vi "Straight line spline generator.vi"(10 "Y":dbl format="%#_13g", 11 "X":dbl format="%#_13g") -> (2 "bx^3":dbl, 3 "ax^3":dbl)   [LabVIEW 2015]
uses:
  <vilib>/Analysis/7linalg.llb/Solve Linear Equations (single right hand).vi
  <vilib>/Analysis/baseanly.llb/Solve Linear Equations By Cholesky.vi
  <vilib>/Analysis/baseanly.llb/Real Matrix to Compact Array.vi
  <vilib>/Analysis/baseanly.llb/Real Compact Tri-Matrix Linear Eqs.vi
  <vilib>/Analysis/7linalg.llb/Solve Linear Eqs (General).vi
  <vilib>/Analysis/7linalg.llb/Solve Linear Eqs (Gen, single right hand).vi
  <vilib>/Analysis/NI_AALPro.lvlib
  Polynomial.vi
  Polynomial First Derivitive.vi
panel:
  out "Y 3":dbl
  out "Y 2":dbl
  out "XY Graph":cluster{dbl[], dbl[]}(graph)
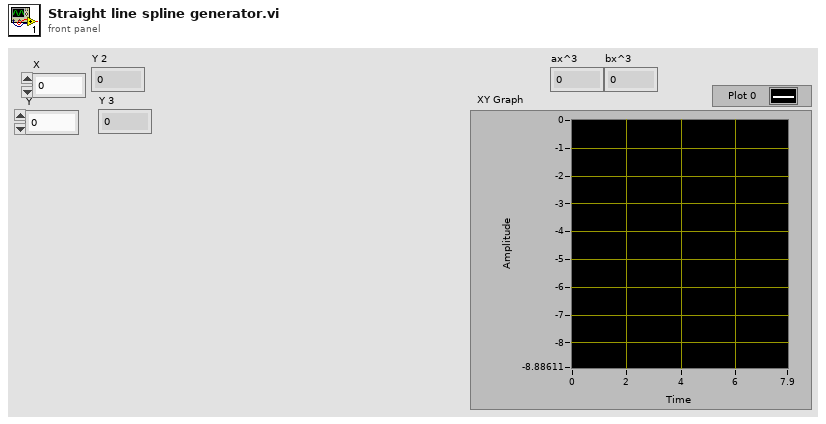
[diagram p1: front panel]
types:
  T1 = typedef "NI_Matrix.lvlib/RealMatrix.ctl" = dbl[][]
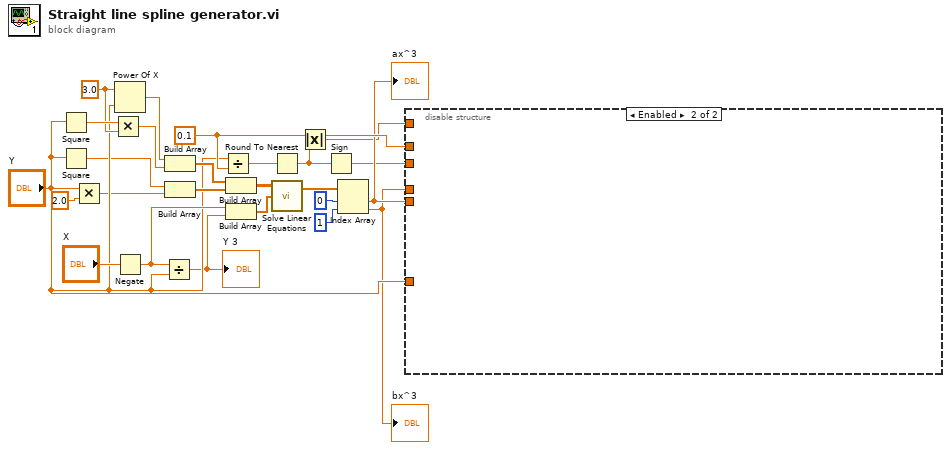
[diagram p0: block diagram]
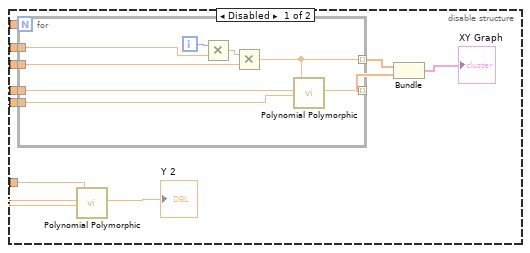
[diagram p2: hidden frame]
diagram:
  w15 = 0.1
  w19 = 3.0 ("y")
  n1 = Square(x="Y") -> (x^2=w20:dbl)
  n2 = Square(x="Y") -> (x^2=w5:dbl)
  n3 = Multiply(x="Y", y=2.0) -> (x*y=w7:dbl)
  n4 = Multiply(x=w20, y=w19) -> (x*y=w8:dbl)
  n5 = Power Of X(1:"Y", 2:w19) -> (0:w6:dbl)
  n6 = Negate(x="X") -> (-x=w14:dbl)
  n7 = Divide(x=w14, y="Y") -> (x/y=w4:dbl)
  "Y 3" <- w4
  n8 = Build Array(w6, w8) -> (w25:dbl[])
  n9 = Build Array(w5, w7) -> (w24:dbl[])
  n10 = Divide(x="Y", y=w15) -> (x/y=w16:dbl)
  n11 = Build Array(w25, w24) -> (w23:T1)
  n12 = Build Array(w14, w4) -> (w21:dbl[])
  n13 = Round To Nearest(number=w16) -> (nearest integer value=w3:dbl)
  n14 = call-poly <vilib>:"Solve Linear Equations.vi"("Known Vector"=w21, "Input Matrix"=w23) -> ("Solution Vector"=w17:dbl[])  [unwired: 1 in, 1 out]
  n15 = Absolute Value(x=w3) -> (abs(x)=w1:dbl)
  n16 = Sign(1:w3) -> (0:w2:dbl)
  n17 = Index Array(array=w17, index #1=0 ("index"), index #2=1 ("index")) -> (element #1=w10:dbl, element #2=w9:dbl)
  "ax^3" <- w10
  "bx^3" <- w9
  n18 = disable-structure shown="Enabled" {
    disable-tunnel: w15 -> [w35 _]
    disable-tunnel: "Y" -> [w32 _]
    disable-tunnel: w10 -> [w30 _]
    disable-tunnel: w9 -> [w29 _]
    disable-tunnel: w2 -> [w28 _]
    disable-tunnel: w1 -> [w26 _]
    frame Disabled {
      n19 = for {
        N: w26 -> [_]
        tunnel: w29 -> [w43]
        tunnel: w30 -> [w42]
        tunnel: w35 -> [w40]
        tunnel: [w39] -> w33 mode=indexing
        tunnel: [w37] -> w27 mode=indexing
        tunnel: w28 -> [w36]
        i -> [w41]
        n20 = Multiply(x=w41, y=w40) -> (x*y=w38:dbl)
        n21 = Multiply(x=w38, y=w36) -> (x*y=w37:dbl)
        n22 = call-poly "Polynomial Polymorphic.vi"("CX^2"=w43, "DX^3"=w42, "X"=w37) -> ("Y"=w39:dbl)  [unwired: 16 in]
      }
      n23 = call-poly "Polynomial Polymorphic.vi"("CX^2"=w29, "DX^3"=w30, "X"=w32) -> ("Y"=→"Y 2":dbl)  [unwired: 16 in]
      n24 = Bundle(w27, w33) -> (→"XY Graph":cluster{dbl[], dbl[]})  [unwired: 1 in]
    }
    frame Enabled {
    }
  }
